vi "Write Icon Data.vi"(8 "error in (no error)":errorcluster, 9 "UI Icon":refnum<class "Icon.lvclass">, 10 "Icon":refnum<class "Icon.lvclass">, 11 "ProjectItem in":refnum<class "ProjectItem.lvclass">) -> (0 "error out":errorcluster, 3 "ProjectItem out":refnum<class "ProjectItem.lvclass">)   [LabVIEW 2019, in "ProjectItem.lvclass"]
uses:
  ProjectItem.lvclass
  <vilib>/LabVIEW Icon API/lv_icon/Classes/Icon/Icon.lvclass
  ProjectItem.lvclass/ProjectItem.ctl
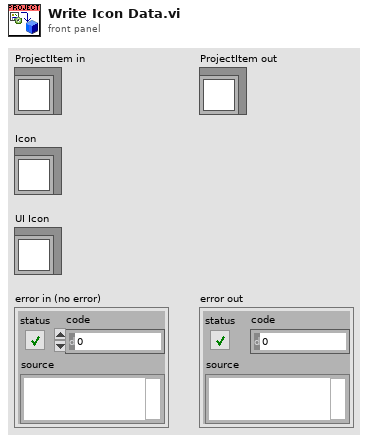
[diagram p1: front panel]
types:
  T1 = cluster{"Class":refnum<vi>, "DynamicVIs":refnum<vi>[], "StaticVIs":refnum<vi>[], "Controls":refnum<vi>[], "Name":string, "Icon":refnum<class "Icon.lvclass">, "Wire Foreground Color":u32}[]
  T2 = cluster{"Class":refnum<vi>, "DynamicVIs":refnum<vi>[], "StaticVIs":refnum<vi>[], "Controls":refnum<vi>[], "Name":string, "Icon":refnum<class "Icon.lvclass">, "Wire Foreground Color":u32}
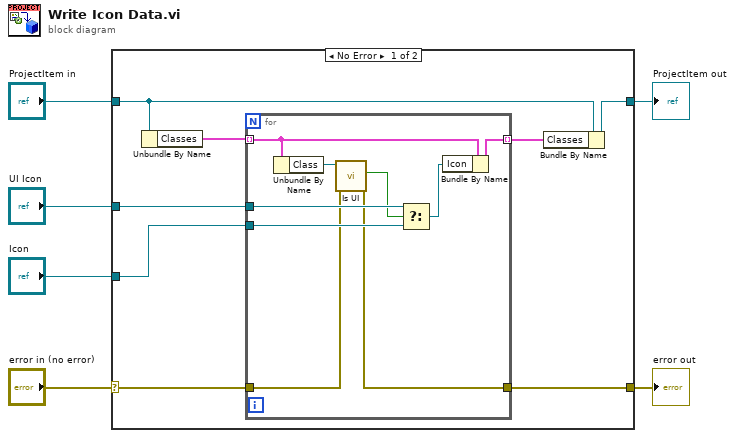
[diagram p0: block diagram]
diagram:
  n1 = case shown="No Error" "error in (no error)" {
    selector: "error in (no error)" -> [w7 w24]
    tunnel: "Icon" -> [w13 _]
    tunnel: "UI Icon" -> [w12 _]
    tunnel: "ProjectItem in" -> [w10 w25]
    tunnel: [w9 w25] -> w3
    tunnel: [w8 w24] -> w2
    frame No Error {
      n2 = Unbundle By Name(w10) -> ("Classes"=w11:T1)
      n3 = for {
        tunnel: w11 -> [w15] mode=indexing
        tunnel: w12 -> [w23]
        tunnel: w13 -> [w22]
        tunnel: [w20] -> w14 mode=indexing
        tunnel: w7 -> [w17]
        tunnel: [w18] -> w8
        n4 = Unbundle By Name(w15) -> ("Class"=w19:refnum<vi>)
        n5 = call "Is UI.vi"("error in (no error)"=w17, "LVClassLibrary in"=w19) -> ("error out"=w18:errorcluster, "UI"=w16:bool)  [unwired: 7 in, 1 out]
        n6 = Select(t=w23, s=w16, f=w22) -> (s? t:f=w21:refnum<class "Icon.lvclass">)
        n7 = Bundle By Name(cluster=w15, "Icon"=w21) -> (w20:T2)
      }
      n8 = Bundle By Name(cluster=w10, "Classes"=w14) -> (w9:refnum<class "ProjectItem.lvclass">)
    }
    frame Error {
    }
  }
  "ProjectItem out" <- w3
  "error out" <- w2
